vi "HAB Climber.vi"   [LabVIEW 2018]
uses:
  <vilib>/Rock Robotics/SystemInterfaces/DIO/FPGA_DIOChannel.ctl
  <vilib>/Rock Robotics/WPI/ThirdParty/Phoenix-LabVIEW/Motor Controller/Controls/CTRE_Phoenix_MotorControl_ControlMode.ctl
  HAB Climber Global.vi
  <vilib>/Rock Robotics/WPI/Switch/WPI_SwitchOpenLimit.vi
  Times/Times Global.vi
  Controllers/Driver Controller/Driver Controller Global.vi
  Cargo Intake/Cargo Intake Global.vi
types:
  T1 = typedef "FPGA_DIOChannel.ctl" = enum8{"DIO 0", "DIO 1", "DIO 2", "DIO 3", "DIO 4", "DIO 5", "DIO 6", "DIO 7", "DIO 8", "DIO 9", "DIO MXP 0", "DIO MXP 1", "DIO MXP 2", "DIO MXP 3", "DIO MXP 4", "DIO MXP 5", "DIO MXP 6", "DIO MXP 7", "DIO MXP 8", "DIO MXP 9", "DIO MXP 10", "DIO MXP 11", "DIO MXP 12", "DIO MXP 13", "DIO MXP 14", "DIO MXP 15", "SPI Port CS1", "SPI Port CS2", "SPI Port CS3", "SPI Port MISO", "SPI Port MOSI", "Invalid"}
  T2 = enum16{"HAB Climber Full Manual Mode", "HAB Climber Manual Mode", "HAB Climber Automated Mode", "HAB Climber Fully Automated Mode"}
  T3 = typedef "WPI_SwitchDevRef.ctl" = cluster{"DevStatus":errorcluster, "DIO Channel":T1, "CntIndex":T4, "Normally Closed":bool}
  T4 = typedef "FPGA_CounterCtrSystemIndex.ctl" = enum8{"Ctr 0", "Ctr 1", "Ctr 2", "Ctr 3", "Ctr 4", "Ctr 5", "Ctr 6", "Ctr 7", "Invalid"}
  T5 = typedef "WPI_MotorControlDeviceRef.ctl" = cluster{"DeviceStatus":errorcluster, "Type":T6, "PWM":cluster{"PWM Channel":T7, "DeadBand":T8}, "CAN":cluster{"Device Number":u8, "SetOutput VI Ref":variant, "GetOutput VI Ref":variant, "Enable VI Ref":variant, "Disable VI Ref":variant, "Data":variant}, "Invert":bool, "DIO PWM":cluster{"PWM \"Enable\" Channel":T7, "DIOChannel":T1, "PWM Rate":dbl}}
  T6 = typedef "WPI_MotorControlType.ctl" = enum16{"PWM", "CAN", "DIO PWM"}
  T7 = typedef "FPGA_DIOPWMChannel.ctl" = enum8{"PWM 0", "PWM 1", "PWM 2", "PWM 3", "PWM 4", "PWM 5", "PWM 6", "PWM 7", "PWM 8", "PWM 9", "PWM MXP 0", "PWM MXP 1", "PWM MXP 2", "PWM MXP 3", "PWM MXP 4", "PWM MXP 5", "PWM MXP 6", "PWM MXP 7", "PWM MXP 8", "PWM MXP 9", "Invalid"}
  T8 = typedef "WPI_PWMDeadband.ctl" = cluster{"Name":string, "maxPositivePwm":i32, "minPositivePwm":i32, "centerPwm":i32, "maxNegativePwm":i32, "minNegativePwm":i32, "angularRange":u16}
  T9 = typedef "Control 3.ctl" = dbl
  T10 = typedef "CTRE_Phoenix_MotorControl_ControlMode.ctl" = u16
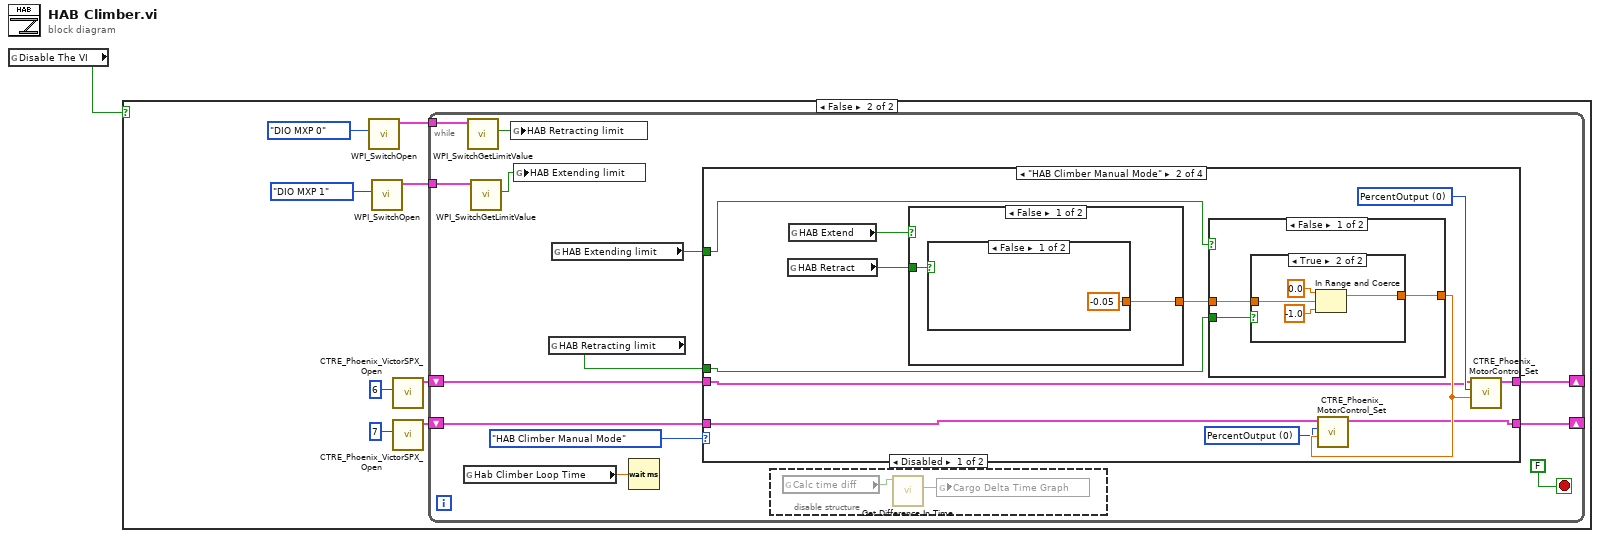
[diagram p0: block diagram]
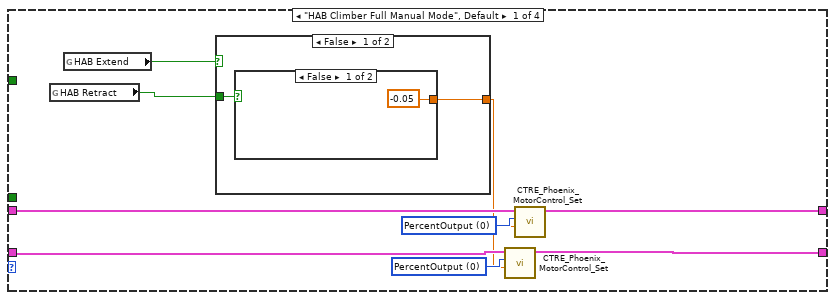
[diagram p4: hidden frame]
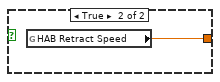
[diagram p5: hidden frame]
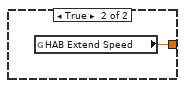
[diagram p6: hidden frame]
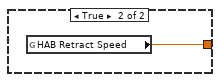
[diagram p7: hidden frame]
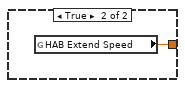
[diagram p8: hidden frame]
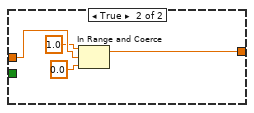
[diagram p10: hidden frame]
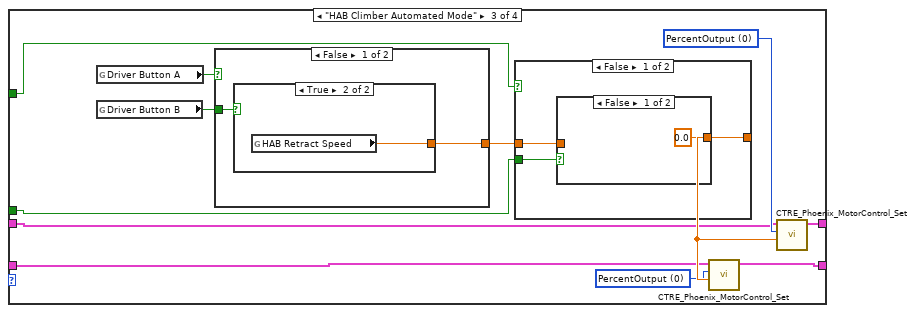
[diagram p11: hidden frame]
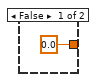
[diagram p12: hidden frame]
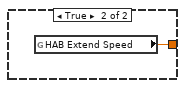
[diagram p13: hidden frame]
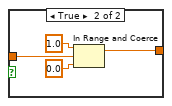
[diagram p14: hidden frame]
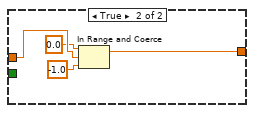
[diagram p15: hidden frame]
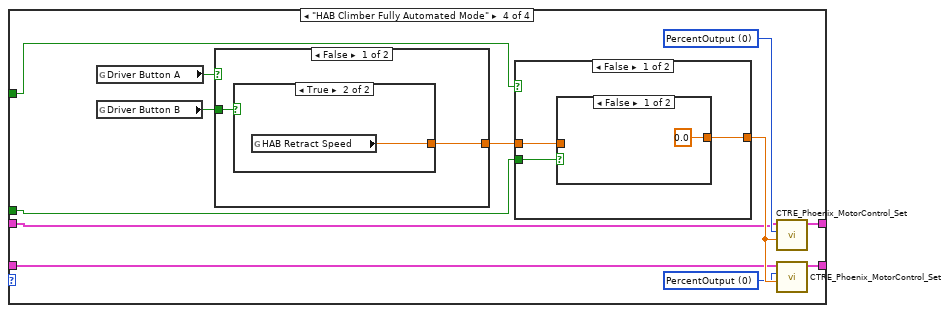
[diagram p16: hidden frame]
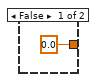
[diagram p17: hidden frame]
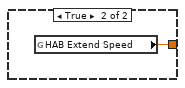
[diagram p18: hidden frame]
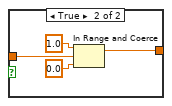
[diagram p19: hidden frame]
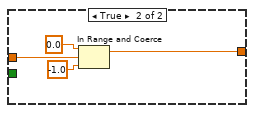
[diagram p20: hidden frame]
diagram:
  n1 = global read "HAB Climber Global.vi" "Disable The VI"() -> (w1:bool)
  n2 = case shown="False" w1 {
    frame True {
    }
    frame False {
      n3 = call-poly <vilib>:"WPI_SwitchOpen.vi"("DIO Channel"=FPGA_DIOChannel."DIO MXP 0") -> ("SwitchDevRef"=w3:T3)  [unwired: 9 in, 1 out]
      n4 = call-poly <vilib>:"WPI_SwitchOpen.vi"("DIO Channel"=FPGA_DIOChannel."DIO MXP 1") -> ("SwitchDevRef"=w2:T3)  [unwired: 9 in, 1 out]
      n5 = call <vilib>:"CTRE_Phoenix_VictorSPX_Open.vi"("Device Number"=u8 6) -> ("CAN Talon SRX Ref"=w9:T5)  [unwired: 9 in, 1 out]
      n6 = call <vilib>:"CTRE_Phoenix_VictorSPX_Open.vi"("Device Number"=u8 7) -> ("CAN Talon SRX Ref"=w7:T5)  [unwired: 9 in, 1 out]
      n7 = while {
        shift-right: [w17] -> _
        shift-left: w9 -> [w19]
        shift-right: [w16] -> _
        shift-left: w7 -> [w18]
        tunnel: w3 -> [w15]
        tunnel: w2 -> [w14]
        stop <- FALSE stop-if-true
        n8 = global read "Times Global.vi" "Hab Climber Loop Time"() -> (w22:T9)
        n9 = call <vilib>:"WPI_SwitchGetLimitValue.vi"("SwitchDevRef"=w15) -> ("Switch Pressed"=w10:bool)  [unwired: 8 in, 2 out]
        n10 = call <vilib>:"WPI_SwitchGetLimitValue.vi"("SwitchDevRef"=w14) -> ("Switch Pressed"=w11:bool)  [unwired: 8 in, 2 out]
        n11 = global write "HAB Climber Global.vi" "HAB Retracting limit"(w10) -> ()
        n12 = global write "HAB Climber Global.vi" "HAB Extending limit"(w11) -> ()
        n13 = global read "HAB Climber Global.vi" "HAB Retracting limit"() -> (w12:bool)
        n14 = global read "HAB Climber Global.vi" "HAB Extending limit"() -> (w13:bool)
        n15 = Wait (ms)(milliseconds to wait=w22) -> ()  [unwired: 1 out]
        n16 = case shown="\"HAB Climber Manual Mode\"" T2."HAB Climber Manual Mode" ("Mode") {
          tunnel: w19 -> [w30 w46 w73 w102]
          tunnel: w18 -> [w31 w45 w72 w101]
          tunnel: [w28 w44 w71 w100] -> w17
          tunnel: [w27 w43 w70 w99] -> w16
          tunnel: w13 -> [_ w42 w69 w98]
          tunnel: w12 -> [_ w41 w68 w97]
          frame "HAB Climber Full Manual Mode", Default {
            w32 = T10 0 items=["PercentOutput"=0, "Position"=1, "Velocity"=2, "Current"=3, "Follower"=5, "MotionProfile"=6, "MotionMagic"=7, "MotionProfileArc"=10, "Disabled"=15] ("Control Mode")
            w33 = T10 0 items=["PercentOutput"=0, "Position"=1, "Velocity"=2, "Current"=3, "Follower"=5, "MotionProfile"=6, "MotionMagic"=7, "MotionProfileArc"=10, "Disabled"=15] ("Control Mode")
            n17 = global read "HAB Climber Global.vi" "HAB Retract"() -> (w25:bool)
            n18 = global read "HAB Climber Global.vi" "HAB Extend"() -> (w26:bool)
            n19 = case shown="False" w26 {
              tunnel: w25 -> [w35 _]
              tunnel: [w34 w38] -> w29
              frame False {
                n20 = case shown="False" w35 {
                  tunnel: [-0.05 w37] -> w34
                  frame False {
                  }
                  frame True {
                    n21 = global read "HAB Climber Global.vi" "HAB Retract Speed"() -> (w37:dbl)
                  }
                }
              }
              frame True {
                n22 = global read "HAB Climber Global.vi" "HAB Extend Speed"() -> (w38:dbl)
              }
            }
            n23 = call <vilib>:"CTRE_Phoenix_MotorControl_Set.vi"("Output"=w29, "Control Mode"=w32, "PhoenixMotorControlDevRef"=w31) -> ("PhoenixMotorControlDevRef"=w27:T5)  [unwired: 7 in, 1 out]
            n24 = call <vilib>:"CTRE_Phoenix_MotorControl_Set.vi"("Output"=w29, "Control Mode"=w33, "PhoenixMotorControlDevRef"=w30) -> ("PhoenixMotorControlDevRef"=w28:T5)  [unwired: 7 in, 1 out]
          }
          frame "HAB Climber Manual Mode" {
            w47 = T10 0 items=["PercentOutput"=0, "Position"=1, "Velocity"=2, "Current"=3, "Follower"=5, "MotionProfile"=6, "MotionMagic"=7, "MotionProfileArc"=10, "Disabled"=15] ("Control Mode")
            w49 = T10 0 items=["PercentOutput"=0, "Position"=1, "Velocity"=2, "Current"=3, "Follower"=5, "MotionProfile"=6, "MotionMagic"=7, "MotionProfileArc"=10, "Disabled"=15] ("Control Mode")
            n25 = global read "HAB Climber Global.vi" "HAB Retract"() -> (w39:bool)
            n26 = global read "HAB Climber Global.vi" "HAB Extend"() -> (w40:bool)
            n27 = case shown="False" w40 {
              tunnel: w39 -> [w52 _]
              tunnel: [w51 w55] -> w50
              frame False {
                n28 = case shown="False" w52 {
                  tunnel: [-0.05 w54] -> w51
                  frame False {
                  }
                  frame True {
                    n29 = global read "HAB Climber Global.vi" "HAB Retract Speed"() -> (w54:dbl)
                  }
                }
              }
              frame True {
                n30 = global read "HAB Climber Global.vi" "HAB Extend Speed"() -> (w55:dbl)
              }
            }
            n31 = case shown="False" w42 {
              tunnel: w50 -> [w57 w67]
              tunnel: [w58 w64] -> w48
              tunnel: w41 -> [w56 _]
              frame False {
                n32 = case shown="True" w56 {
                  tunnel: [w59 w63] -> w58
                  tunnel: w57 -> [w59 w62]
                  frame False {
                  }
                  frame True {
                    n33 = In Range and Coerce(upper limit=0.0, x=w62, lower limit=-1.0) -> (coerced(x)=w63:dbl)  [unwired: 1 out]
                  }
                }
              }
              frame True {
                n34 = In Range and Coerce(upper limit=1.0, x=w67, lower limit=0.0) -> (coerced(x)=w64:dbl)  [unwired: 1 out]
              }
            }
            n35 = call <vilib>:"CTRE_Phoenix_MotorControl_Set.vi"("Output"=w48, "Control Mode"=w47, "PhoenixMotorControlDevRef"=w45) -> ("PhoenixMotorControlDevRef"=w43:T5)  [unwired: 7 in, 1 out]
            n36 = call <vilib>:"CTRE_Phoenix_MotorControl_Set.vi"("Output"=w48, "Control Mode"=w49, "PhoenixMotorControlDevRef"=w46) -> ("PhoenixMotorControlDevRef"=w44:T5)  [unwired: 7 in, 1 out]
          }
          frame "HAB Climber Automated Mode" {
            w74 = T10 0 items=["PercentOutput"=0, "Position"=1, "Velocity"=2, "Current"=3, "Follower"=5, "MotionProfile"=6, "MotionMagic"=7, "MotionProfileArc"=10, "Disabled"=15] ("Control Mode")
            w75 = T10 0 items=["PercentOutput"=0, "Position"=1, "Velocity"=2, "Current"=3, "Follower"=5, "MotionProfile"=6, "MotionMagic"=7, "MotionProfileArc"=10, "Disabled"=15] ("Control Mode")
            n37 = global read "Driver Controller Global.vi" "Driver Button A"() -> (w77:bool)
            n38 = global read "Driver Controller Global.vi" "Driver Button B"() -> (w76:bool)
            n39 = case shown="False" w77 {
              tunnel: w76 -> [w81 _]
              tunnel: [w80 w84] -> w78
              frame False {
                n40 = case shown="True" w81 {
                  tunnel: [0.0 w83] -> w80
                  frame False {
                  }
                  frame True {
                    n41 = global read "HAB Climber Global.vi" "HAB Retract Speed"() -> (w83:dbl)
                  }
                }
              }
              frame True {
                n42 = global read "HAB Climber Global.vi" "HAB Extend Speed"() -> (w84:dbl)
              }
            }
            n43 = case shown="False" w69 {
              tunnel: w78 -> [w86 w96]
              tunnel: [w87 w93] -> w79
              tunnel: w68 -> [w85 _]
              frame False {
                n44 = case shown="False" w85 {
                  tunnel: [0.0 w92] -> w87
                  tunnel: w86 -> [_ w91]
                  frame False {
                  }
                  frame True {
                    n45 = In Range and Coerce(upper limit=1.0, x=w91, lower limit=0.0) -> (coerced(x)=w92:dbl)  [unwired: 1 out]
                  }
                }
              }
              frame True {
                n46 = In Range and Coerce(upper limit=0.0, x=w96, lower limit=-1.0) -> (coerced(x)=w93:dbl)  [unwired: 1 out]
              }
            }
            n47 = call <vilib>:"CTRE_Phoenix_MotorControl_Set.vi"("Output"=w79, "Control Mode"=w74, "PhoenixMotorControlDevRef"=w72) -> ("PhoenixMotorControlDevRef"=w70:T5)  [unwired: 7 in, 1 out]
            n48 = call <vilib>:"CTRE_Phoenix_MotorControl_Set.vi"("Output"=w79, "Control Mode"=w75, "PhoenixMotorControlDevRef"=w73) -> ("PhoenixMotorControlDevRef"=w71:T5)  [unwired: 7 in, 1 out]
          }
          frame "HAB Climber Fully Automated Mode" {
            w103 = T10 0 items=["PercentOutput"=0, "Position"=1, "Velocity"=2, "Current"=3, "Follower"=5, "MotionProfile"=6, "MotionMagic"=7, "MotionProfileArc"=10, "Disabled"=15] ("Control Mode")
            w104 = T10 0 items=["PercentOutput"=0, "Position"=1, "Velocity"=2, "Current"=3, "Follower"=5, "MotionProfile"=6, "MotionMagic"=7, "MotionProfileArc"=10, "Disabled"=15] ("Control Mode")
            n49 = global read "Driver Controller Global.vi" "Driver Button A"() -> (w106:bool)
            n50 = global read "Driver Controller Global.vi" "Driver Button B"() -> (w105:bool)
            n51 = case shown="False" w106 {
              tunnel: w105 -> [w110 _]
              tunnel: [w109 w113] -> w107
              frame False {
                n52 = case shown="True" w110 {
                  tunnel: [0.0 w112] -> w109
                  frame False {
                  }
                  frame True {
                    n53 = global read "HAB Climber Global.vi" "HAB Retract Speed"() -> (w112:dbl)
                  }
                }
              }
              frame True {
                n54 = global read "HAB Climber Global.vi" "HAB Extend Speed"() -> (w113:dbl)
              }
            }
            n55 = case shown="False" w98 {
              tunnel: w107 -> [w115 w125]
              tunnel: [w116 w122] -> w108
              tunnel: w97 -> [w114 _]
              frame False {
                n56 = case shown="False" w114 {
                  tunnel: [0.0 w121] -> w116
                  tunnel: w115 -> [_ w120]
                  frame False {
                  }
                  frame True {
                    n57 = In Range and Coerce(upper limit=1.0, x=w120, lower limit=0.0) -> (coerced(x)=w121:dbl)  [unwired: 1 out]
                  }
                }
              }
              frame True {
                n58 = In Range and Coerce(upper limit=0.0, x=w125, lower limit=-1.0) -> (coerced(x)=w122:dbl)  [unwired: 1 out]
              }
            }
            n59 = call <vilib>:"CTRE_Phoenix_MotorControl_Set.vi"("Output"=w108, "Control Mode"=w104, "PhoenixMotorControlDevRef"=w102) -> ("PhoenixMotorControlDevRef"=w100:T5)  [unwired: 7 in, 1 out]
            n60 = call <vilib>:"CTRE_Phoenix_MotorControl_Set.vi"("Output"=w108, "Control Mode"=w103, "PhoenixMotorControlDevRef"=w101) -> ("PhoenixMotorControlDevRef"=w99:T5)  [unwired: 7 in, 1 out]
          }
        }
        n61 = disable-structure shown="Disabled" {
          frame Disabled {
            n62 = global read "Cargo Intake Global.vi" "Calc time diff"() -> (w24:bool)
            n63 = call "Get Difference In Time.vi"("Calculate Time Difference"=w24) -> ("Delta Time over Time"=w23:u32)  [unwired: 9 in, 1 out]
            n64 = global write "Times Global.vi" "Cargo Delta Time Graph"(w23) -> ()
          }
          frame Enabled {
          }
        }
      }
    }
  }
